vi "daq.vi"() -> ()   [LabVIEW 2015]
uses:
  <vilib>/DAQmx/write.llb/DAQmx Write (Analog 1D Wfm NChan NSamp).vi
  <vilib>/DAQmx/read.llb/DAQmx Read (Analog 1D Wfm NChan NSamp).vi
  <vilib>/DAQmx/create/channels.llb/DAQmx Create Channel (AI-Voltage-Basic).vi
  <vilib>/DAQmx/configure/timing.llb/DAQmx Timing (Sample Clock).vi
  <vilib>/DAQmx/miscellaneous.llb/DAQmx Fill In Error Info.vi
  <vilib>/DAQmx/create/channels.llb/DAQmx Create Channel (AO-Voltage-Basic).vi
  <vilib>/express/express analysis/Spectral/Block/exnSpectralBlock spectral measurements RMS poly.vi
  <vilib>/express/express analysis/Spectral/Block/exnSpectralBlock spectral measurements RMS array WFM.vi
  <vilib>/express/express analysis/Spectral/XNode/ExpressSpectralMeasurementsBlockNode.xnode
  <resource>/objmgr/daqmx.rc
panel:
  out "SampClk.Rate":dbl
  out "Waveform Graph 2":cluster{"f0":dbl, "df":dbl, "magnitude":dbl[]}[](graph)
  out "Waveform Graph":waveform(dbl)[](graph)
  out "error out":errorcluster
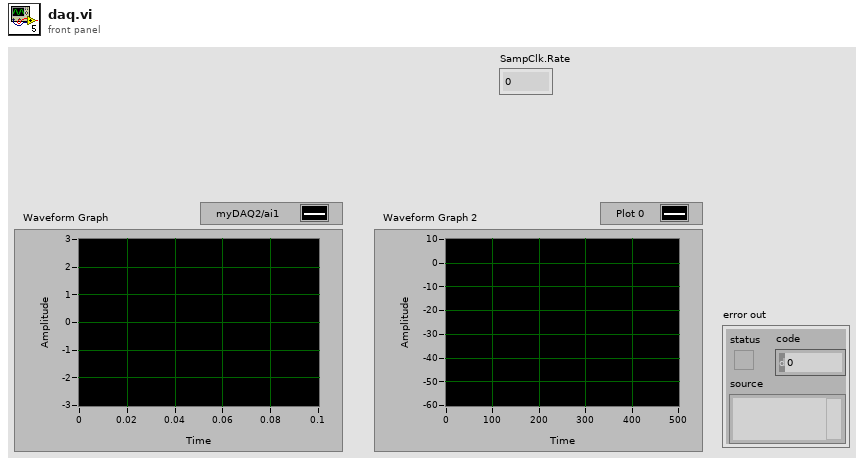
[diagram p1: front panel]
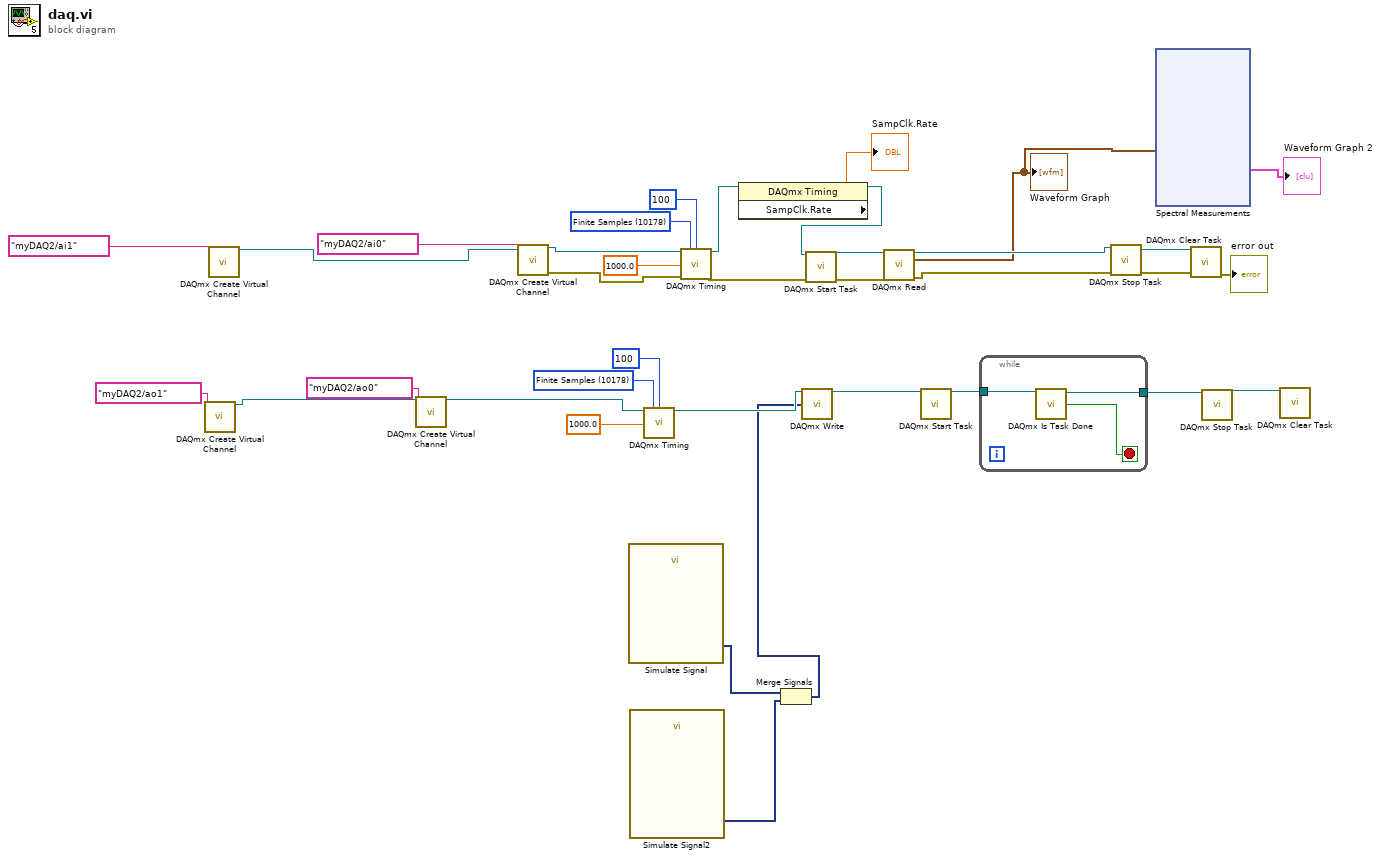
[diagram p0: block diagram]
diagram:
  w14 = 10178 items=["Finite Samples"=10178, "Continuous Samples"=10123, "Hardware Timed Single Point"=12522] ("sample mode")
  w33 = 10178 items=["Finite Samples"=10178, "Continuous Samples"=10123, "Hardware Timed Single Point"=12522] ("sample mode")
  n1 = call-poly <vilib>:"DAQmx Create Virtual Channel.vi"("physical channels"=tag "myDAQ2/ao1") -> ("task out"=w16:refnum<k21>)  [unwired: 13 in, 1 out]
  n2 = call-poly <vilib>:"DAQmx Create Virtual Channel.vi"("physical channels"=tag "myDAQ2/ai1") -> ("task out"=w21:refnum<k21>)  [unwired: 13 in, 1 out]
  n3 = call-poly <vilib>:"DAQmx Create Virtual Channel.vi"("task in"=w16, "physical channels"=tag "myDAQ2/ao0") -> ("task out"=w12:refnum<k21>)  [unwired: 12 in, 1 out]
  n4 = call-poly <vilib>:"DAQmx Create Virtual Channel.vi"("task in"=w21, "physical channels"=tag "myDAQ2/ai0") -> ("task out"=w35:refnum<k21>, "error out"=w29:errorcluster)  [unwired: 12 in]
  n5 = call "Simulate Signal"() -> ("Sine"=w10:dynamicdata)  [unwired: 14 in, 1 out]
  n6 = call "Simulate Signal2"() -> ("Square"=w9:dynamicdata)  [unwired: 14 in, 1 out]
  n7 = call-poly <vilib>:"DAQmx Timing.vi"("task/channels in"=w12, "sample mode"=w14, "samples per channel"=100, "rate"=1000.0) -> ("task out"=w11:refnum<k21>)  [unwired: 10 in, 1 out]
  n8 = call-poly <vilib>:"DAQmx Timing.vi"("task/channels in"=w35, "sample mode"=w33, "samples per channel"=100, "rate"=1000.0, "error in"=w29) -> ("task out"=w3:refnum<k21>, "error out"=w28:errorcluster)  [unwired: 9 in]
  n9 = property class="DAQmx Timing"(reference=w3) -> (reference out=w2:refnum<k21>, "SampClk.Rate"=→"SampClk.Rate":dbl)  [unwired: 1 in, 1 out]
  n10 = Merge Signals(w10, w9) -> (w8:dynamicdata)
  n11 = call-poly <vilib>:"DAQmx Write.vi"("task/channels in"=w11, "data"=w8) -> ("task out"=w7:refnum<k21>)  [unwired: 11 in, 2 out]
  n12 = call <vilib>:"DAQmx Start Task.vi"("task/channels in"=w2, "error in"=w28) -> ("task out"=w24:refnum<k21>, "error out"=w23:errorcluster)  [unwired: 12 in]
  n13 = call-poly <vilib>:"DAQmx Read.vi"("task/channels in"=w24, "error in"=w23) -> ("task out"=w31:refnum<k21>, "data"=w20:waveform(dbl)[], "error out"=w27:errorcluster)  [unwired: 11 in]
  "Waveform Graph" <- w20
  n14 = call <vilib>:"DAQmx Start Task.vi"("task/channels in"=w7) -> ("task out"=w6:refnum<k21>)  [unwired: 13 in, 1 out]
  n15 = while {
    tunnel: w6 -> [w38]
    tunnel: [w37] -> w5
    stop <- w39 stop-if-true
    n16 = call <vilib>:"DAQmx Is Task Done.vi"("task/channels in"=w38) -> ("task out"=w37:refnum<k21>, "task done?"=w39:bool)  [unwired: 12 in, 1 out]
  }
  n17 = call <vilib>:"DAQmx Stop Task.vi"("task/channels in"=w31, "error in"=w27) -> ("task out"=w30:refnum<k21>, "error out"=w26:errorcluster)  [unwired: 12 in]
  n18 = xnode "Spectral Measurements"("Signals"=w20) -> ("FFT - (RMS)"=→"Waveform Graph 2":cluster{"f0":dbl, "df":dbl, "magnitude":dbl[]}[])  [unwired: 1 in, 2 out]
  n19 = call <vilib>:"DAQmx Clear Task.vi"("task in"=w30, "error in"=w26) -> ("error out"=→"error out":errorcluster)  [unwired: 13 in]
  n20 = call <vilib>:"DAQmx Stop Task.vi"("task/channels in"=w5) -> ("task out"=w4:refnum<k21>)  [unwired: 13 in, 1 out]
  n21 = call <vilib>:"DAQmx Clear Task.vi"("task in"=w4) -> ()  [unwired: 14 in, 1 out]
